vi "from var.vi"(11 "Queue in":refnum<queue>) -> (2 "data jazda":T1 {"Data"."array of cans"."type" items=["CAN Data", "CAN Remote"]; "Data"."array of cans"."identifier" format="%.0x"}, 3 "data konfig":cluster{"bool":bool, "ramki konf":T2} {"ramki konf"."type" items=["CAN Data", "CAN Remote"]; "ramki konf"."identifier" format="%.0x"})   [LabVIEW 2015]
uses:
  <vilib>/RioEmbeddedCAN/RioEmbeddedCAN.llb/CANFrameControl.ctl
  PC/QMH Fundamentals - Message Cluster.ctl
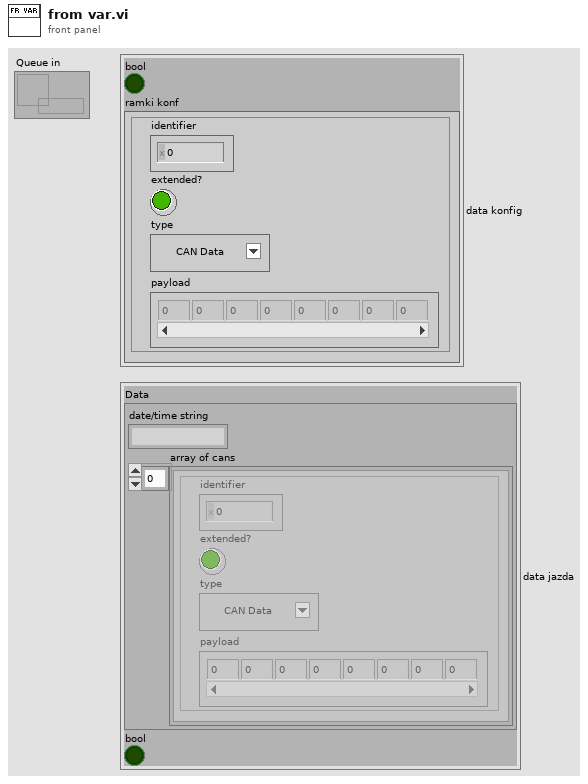
[diagram p1: front panel]
types:
  T1 = cluster{"Data":cluster{"date/time string":string, "array of cans":cluster{"identifier":u32, "extended?":bool, "type":u8, "payload":u8[]}[]}, "bool":bool}
  T2 = typedef "CANFrameControl.ctl" = cluster{"identifier":u32, "extended?":bool, "type":u8, "payload":i8[]}
  T3 = typedef "QMH Fundamentals - Message Cluster.ctl" = cluster{"Message":string, "Message Data":variant}
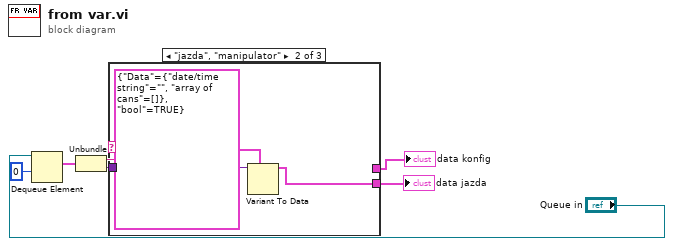
[diagram p0: block diagram]
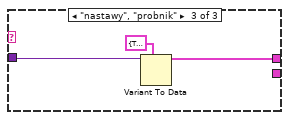
[diagram p3: hidden frame]
diagram:
  n1 = Dequeue Element(queue="Queue in", timeout in ms (-1)=0) -> (element=w3:T3)  [unwired: 1 in, 3 out]
  n2 = Unbundle(w3) -> ("Message"=w4:string, "Message Data"=w5:variant)
  n3 = case shown="\"jazda\", \"manipulator\"" w4 {
    tunnel: w5 -> [_ w9 w12]
    tunnel: [_ _ w11] -> w6
    tunnel: [_ w8 _] -> w7
    frame "nothing", Default {
    }
    frame "jazda", "manipulator" {
      n4 = Variant To Data(type=T1 {"Data"={"date/time string"="", "array of cans"=[]}, "bool"=TRUE} ("jazda"), Variant=w9) -> (data=w8:T1)  [unwired: 1 in, 1 out]
    }
    frame "nastawy", "probnik" {
      n5 = Variant To Data(type=cluster{"bool":bool, "ramki konf":T2} {"bool"=TRUE, "ramki konf"={"identifier"=0, "extended?"=TRUE, "type"=1, "payload"=[]}} ("jazda"), Variant=w12) -> (data=w11:cluster{"bool":bool, "ramki konf":T2})  [unwired: 1 in, 1 out]
    }
  }
  "data konfig" <- w6
  "data jazda" <- w7
